vi "GetText.vi"(8 "error in":errorcluster, 11 "EthernetIP editor node in":refnum<class "EIP Tags editor node.lvclass">) -> (0 "error out":errorcluster, 1 "additional text":string, 2 "text":string, 3 "EthernetIP editor node out":refnum<class "EIP Tags editor node.lvclass">, 4 "glyph":string)   [LabVIEW 2013, in "EIP Tags editor node.lvclass"]
uses:
  EIP Tags editor node.lvclass
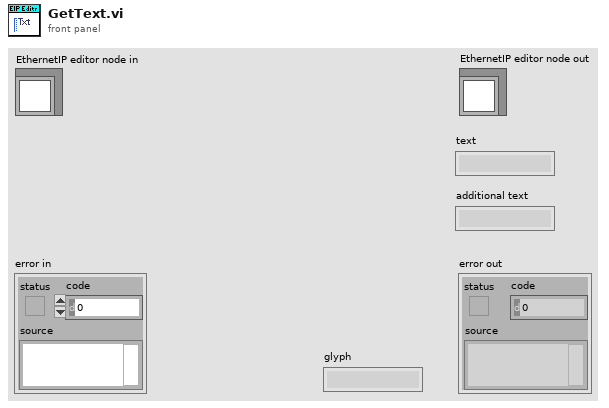
[diagram p1: front panel]
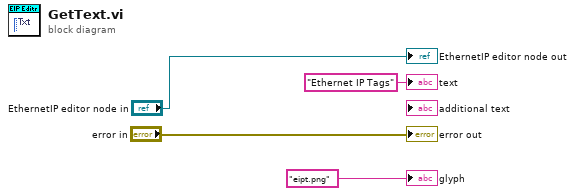
[diagram p0: block diagram]
diagram:
  "error out" <- "error in"
  "EthernetIP editor node out" <- "EthernetIP editor node in"
  "text" <- "Ethernet IP Tags" ("text")
  "glyph" <- "eipt.png" ("glyph")
